vi "_Init UI.vi"(8 "error in (no error)":errorcluster, 10 "Type":T1, 11 "UI_ProgressDlg in":refnum<class "UI_ProgressDlg.lvclass">) -> (0 "error out":errorcluster, 3 "UI_ProgressDlg out":refnum<class "UI_ProgressDlg.lvclass">)   [LabVIEW 2014, in "UI_ProgressDlg.lvlib" / "UI_ProgressDlg.lvclass"]
uses:
  UI_ProgressDlg.lvclass
  _Control/DEF-Type.ctl
  UI_ProgressDlg.lvclass/UI_ProgressDlg.ctl
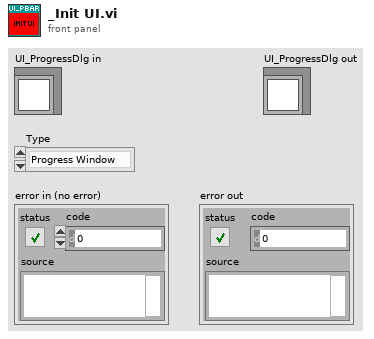
[diagram p1: front panel]
types:
  T1 = typedef "UI_ProgressDlg.lvlib/UI_ProgressDlg.lvclass/DEF-Type.ctl" = enum16{"Progress Window", "Buzy Window", "Timer Window"}
  T2 = enum32{"Invalid", "Standard", "Closed", "Hidden", "Minimized", "Maximized"}
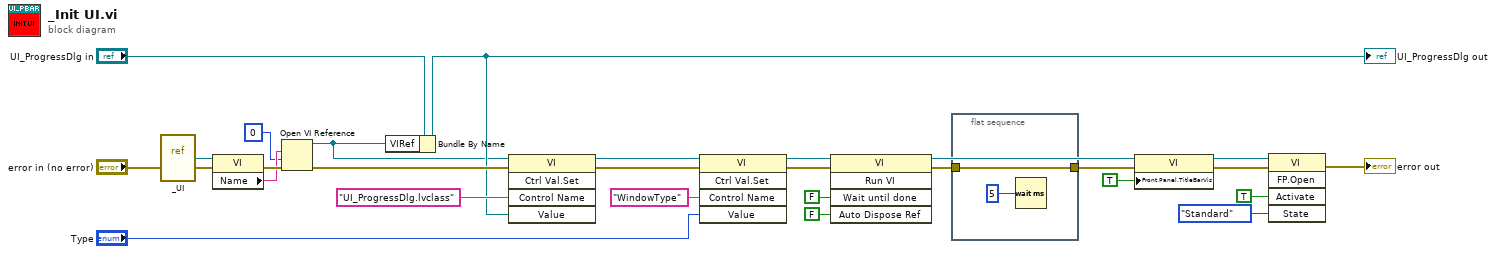
[diagram p0: block diagram]
diagram:
  n1 = vi-ref "_UI.vi"() -> (w19:refnum<vi>)
  n2 = property on="Property Node" class="VI"(reference=w19, error in="error in (no error)") -> (error out=w7:errorcluster, "Name"=w6:string)  [unwired: 1 out]
  n3 = Open VI Reference(vi path=w6, options=0, error in (no error)=w7) -> (vi reference=w1:refnum<vi>, error out=w4:errorcluster)  [unwired: 3 in]
  n4 = Bundle By Name(cluster="UI_ProgressDlg in", "VIRef"=w1) -> (w2:refnum<class "UI_ProgressDlg.lvclass">)
  "UI_ProgressDlg out" <- w2
  n5 = invoke on="Invoke Node" class="VI" method="Ctrl Val.Set"(reference=w1, error in=w4, "Control Name"="UI_ProgressDlg.lvclass", "Value"=w2) -> (reference out=w20:refnum<vi>, error out=w21:errorcluster)  [unwired: 1 in, 3 out]
  n6 = invoke on="Invoke Node" class="VI" method="Ctrl Val.Set"(reference=w20, error in=w21, "Control Name"="WindowType", "Value"="Type") -> (reference out=w23:refnum<vi>, error out=w22:errorcluster)  [unwired: 1 in, 3 out]
  n7 = invoke on="Invoke Node" class="VI" method="Run VI"(reference=w23, error in=w22, "Wait until done"=FALSE ("Auto Dispose Reference"), "Auto Dispose Ref"=FALSE ("Auto Dispose Reference")) -> (reference out=w11:refnum<vi>, error out=w10:errorcluster)  [unwired: 1 in, 3 out]
  n8 = flat-sequence {
    tunnel: [w29] -> w12
    tunnel: w10 -> [w29]
    frame #0 {
      n9 = Wait (ms)(milliseconds to wait=u32 5) -> ()  [unwired: 1 out]
    }
  }
  n10 = property on="Property Node" class="VI"(reference=w11, error in=w12, "Front Panel.TitleBarVis"=TRUE ("Front Panel Window:Title Bar Visible")) -> (reference out=w15:refnum<vi>, error out=w16:errorcluster)
  n11 = invoke on="Invoke Node" class="VI" method="FP.Open"(reference=w15, error in=w16, "Activate"=TRUE ("Activate?"), "State"=T2."Standard" ("Front Panel Window:State")) -> (error out=→"error out":errorcluster)  [unwired: 1 in, 4 out]
